vi "Stop Core.vi"(10 "final error code":i32, 11 "ViewableActor in":refnum<class "ViewableActor.lvclass">) -> (3 "ViewableActor out":refnum<class "ViewableActor.lvclass">)   [LabVIEW 2012, in "Win8uiFramework.lvlib" / "ViewableActor.lvclass"]
doc: "(<B>Filename</B>: Actor Framework.lvlib:Actor.lvclass:Stop Core.vi)\n\nDefines what the actor does before it stops. Use the <B>final error code</B> input to determine whether the actor shut down in response to an error.\n\nBy default, this method does nothing. A descendant class may override it to define behavior, such as shutting down any processes the actor initiated in its override of the Actor Core method."
uses:
  ViewableActor.lvclass
  ViewableActor.lvclass/ViewableActor.ctl
  <vilib>/ActorFramework/Actor/Actor.lvclass
  Read Stop Event.vi
  Read SubPanel Ref.vi
  Win8uiFramework.lvlib
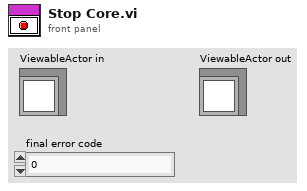
[diagram p1: front panel]
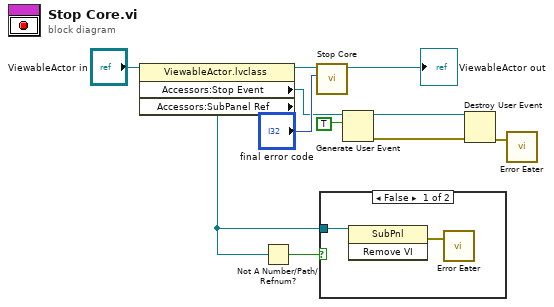
[diagram p0: block diagram]
diagram:
  n1 = property class="ViewableActor.lvclass"(reference="ViewableActor in") -> (reference out=w8:refnum<class "ViewableActor.lvclass">, "Accessors:Stop Event"=w7:refnum<user-event>, "Accessors:SubPanel Ref"=w2:refnum<vi>)  [unwired: 1 in, 1 out]
  n2 = Not A Number/Path/Refnum?(number/path/refnum=w2) -> (NaN/Path/Refnum?=w3:bool)
  n3 = call-parent "Stop Core.vi"("final error code"="final error code", "Actor in"=w8) -> ("Actor out"=→"ViewableActor out":refnum<class "ViewableActor.lvclass">)  [unwired: 9 in]
  n4 = case shown="False" w3 {
    tunnel: w2 -> [w13 _]
    frame False {
      n5 = invoke class="SubPnl" method="Remove VI"(reference=w13) -> (error out=w12:errorcluster)  [unwired: 2 in, 2 out]
      n6 = call "Error Eater.vi"("error in (no error)"=w12) -> ()  [unwired: 2 in]
    }
    frame True {
    }
  }
  n7 = Generate User Event(user event=w7, event data cluster=TRUE ("event data")) -> (user event out=w5:refnum<user-event>, error out=w4:errorcluster)  [unwired: 1 in]
  n8 = Destroy User Event(user event=w5, error in=w4) -> (error out=w1:errorcluster)
  n9 = call "Error Eater.vi"("error in (no error)"=w1) -> ()  [unwired: 2 in]
